vi "Generate Report.vi"(8 "error in (no error)":errorcluster, 11 "Protocol Verification Test in":refnum<class "Protocol Verification Test.lvclass">) -> (0 "error out":errorcluster, 3 "Protocol Verification Test out":refnum<class "Protocol Verification Test.lvclass">)   [LabVIEW 2017, in "Protocol Verification Test.lvlib" / "Protocol Verification Test.lvclass"]
uses:
  Protocol Verification Test.lvclass
  Protocol Verification Test.lvclass/Protocol Verification Test.ctl
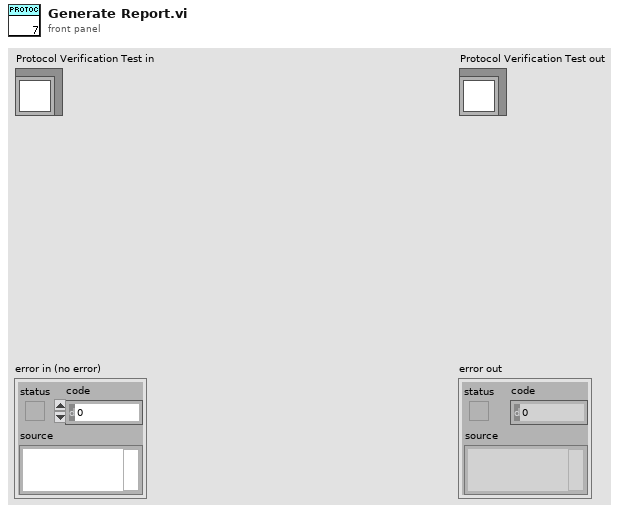
[diagram p1: front panel]
types:
  T1 = typedef "Paths.ctl" = cluster{"Data Directory":path, "Test Config Dir":path, "Error Logs":path, "Event Logs":path, "Settings.Json":path, "Reports Directory":path}
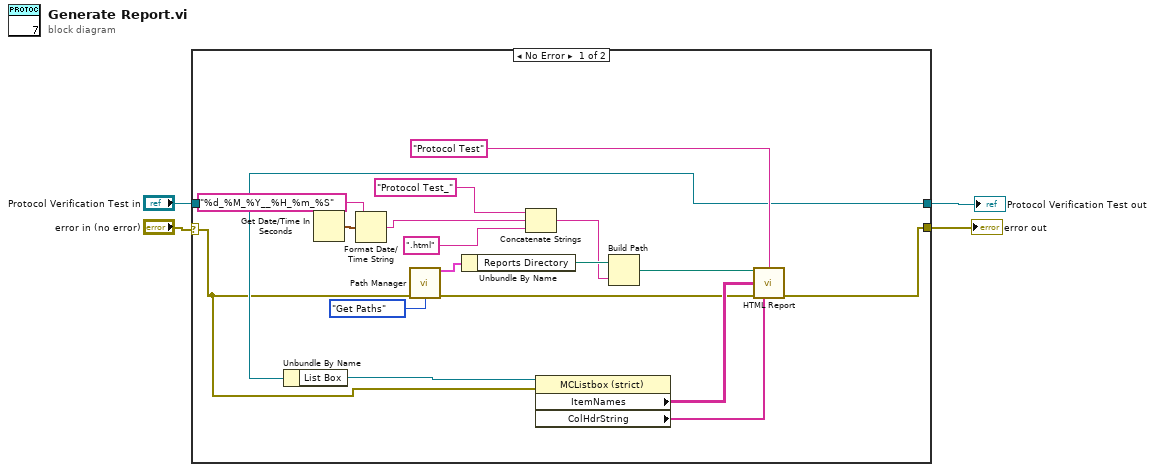
[diagram p0: block diagram]
diagram:
  n1 = case shown="No Error" "error in (no error)" {
    selector: "error in (no error)" -> [w8 w23]
    tunnel: "Protocol Verification Test in" -> [w11 w24]
    tunnel: [w11 w24] -> w2
    tunnel: [w12 w23] -> w1
    frame No Error {
      n2 = Unbundle By Name(w11) -> ("List Box"=w10:refnum<vi>)
      n3 = Get Date/Time In Seconds() -> (seconds since 1Jan1904=w7:timestamp)
      n4 = Format Date/Time String(time format string (%c)="%d_%M_%Y__%H_%m_%S", seconds (now)=w7) -> (date/time string=w5:string)  [unwired: 1 in]
      n5 = call "Path Manager.vi"("Error in (no error)"=w8, "Options"=enum16{"Get Paths", "Init Paths"}."Get Paths") -> ("Cluster"=w22:T1, "Error out"=w13:errorcluster)  [unwired: 12 in]
      n6 = Unbundle By Name(w22) -> ("Reports Directory"=w20:path)
      n7 = Concatenate Strings("Protocol Test_", w5, ".html" ("string")) -> (w19:string)
      n8 = property class="MCListbox (strict)"(reference=w10, error in=w8) -> ("ItemNames"=w16:string[][], "ColHdrString"=w15:string[])  [unwired: 2 out]
      n9 = Build Path(base path=w20, name or relative path=w19) -> (appended path=w18:path)
      n10 = call "HTML Report.vi"("report file path"=w18, "Column Headers"=w15, "Header"="Protocol Test", "Table Data"=w16, "error in (no error)"=w13) -> ("error out"=w12:errorcluster)  [unwired: 10 in]
    }
    frame Error {
    }
  }
  "error out" <- w1
  "Protocol Verification Test out" <- w2
